vi "FITS_WriteImageI32.vi"(6 "Array":i32[](array[numeric])=[0, 0, 0, 0, 0, 0, 0, 0, 0, 0, 0, 0, 0, 0, 0, 0, 0, 0, 0, 0, 0, 0, 0, 0, 0, 0, 0, 0, 0, 0, 0, 0, 0, 0, 0, 0, 0, 0, 0, 0, 0, 0, 0, 0, 0, 0, 0, 0, 0, 0, 0, 0, 0, 0, 0, 1, 0, 0, 0, 0], 7 "ref":u64, 8 "error in":errorcluster, 9 "nelem":i32, 10 "firstel":i32) -> (0 "error out":errorcluster, 2 "result":i32)   [LabVIEW 2016]
uses:
  usr/local/lib/libfits.so
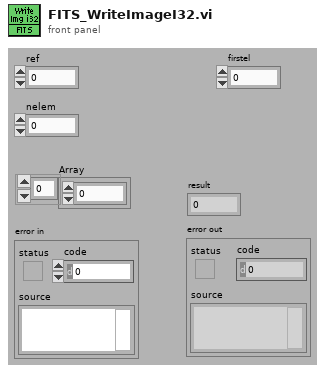
[diagram p1: front panel]
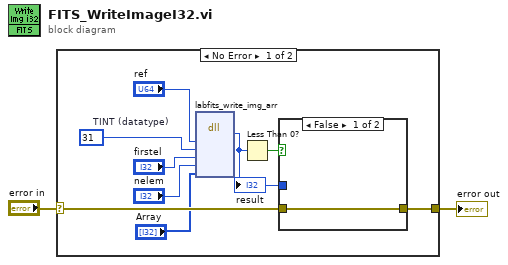
[diagram p0: block diagram]
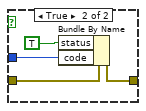
[diagram p2: hidden frame]
diagram:
  n1 = case shown="No Error" "error in" {
    selector: "error in" -> [w10 w17]
    tunnel: [w9 w17] -> w1
    frame No Error {
      w4 = 31  # TINT (datatype)
      n2 = dll-call lib="usr/local/lib/libfits.so" fn="labfits_write_img_arr"("ref"="ref", "datatype"=w4, "firstel"="firstel", "nelem"="nelem", "data_array"="Array") -> ("return type"=w7:i32)  [unwired: 8 in, 2 out]
      "result" <- w7
      n3 = Less Than 0?(x=w7) -> (x < 0?=w11:bool)
      n4 = case shown="False" w11 {
        tunnel: w10 -> [w12 w14]
        tunnel: [w12 w13] -> w9
        tunnel: w7 -> [_ w15]
        frame False {
        }
        frame True {
          n5 = Bundle By Name(cluster=w14, "status"=TRUE, "code"=w15) -> (w13:errorcluster)
        }
      }
    }
    frame Error {
    }
  }
  "error out" <- w1
